vi "TP 1(SubVI).vi"(11 "HT LOC":u64[](array[numeric])) -> ()   [LabVIEW 2015]
panel:
  out "Array 2":T1(array[cluster])
  out "Array":T1(array[cluster])
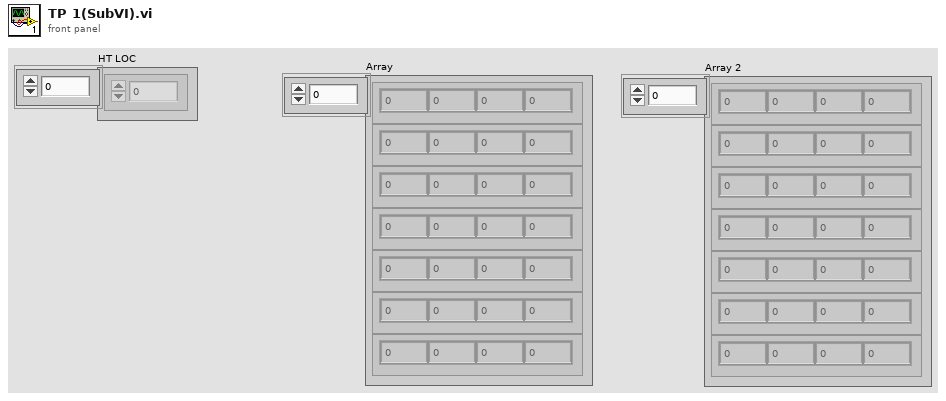
[diagram p1: front panel]
types:
  T1 = cluster{"Numeric Control":u16, "Numeric Control":u16, "Numeric Control":u16, "Numeric Control":u16}[]
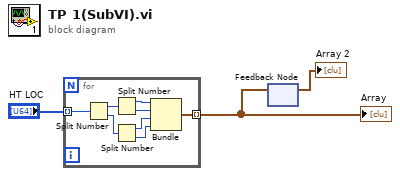
[diagram p0: block diagram]
diagram:
  n1 = for {
    tunnel: "HT LOC" -> [w11] mode=indexing
    tunnel: [w4] -> w2 mode=indexing
    n2 = Split Number(x=w11) -> (hi(x)=w10:u32, lo(x)=w9:u32)
    n3 = Split Number(x=w10) -> (hi(x)=w8:u16, lo(x)=w7:u16)
    n4 = Split Number(x=w9) -> (hi(x)=w6:u16, lo(x)=w5:u16)
    n5 = Bundle(w8, w7, w6, w5) -> (w4:cluster{u16, u16, u16, u16})  [unwired: 1 in]
  }
  "Array" <- w2
  n6 = feedback-in #1(w2) -> ()
  n7 = feedback #1() -> (→"Array 2":cluster{u16, u16, u16, u16}[])  [unwired: 1 in]
